vi "Send Command.vi"(8 "error in (no error)":errorcluster, 10 "command":string, 11 "GH2 in":refnum<class "GH2.lvclass">) -> (0 "error out":errorcluster, 2 "response":string, 3 "GH2 out":refnum<class "GH2.lvclass">)   [LabVIEW 2026, in "GH2.lvclass"]
uses:
  GH2.lvclass
  GH2.lvclass/GH2.ctl
  <vilib>/Utility/error.llb/Trim Whitespace One-Sided.vi
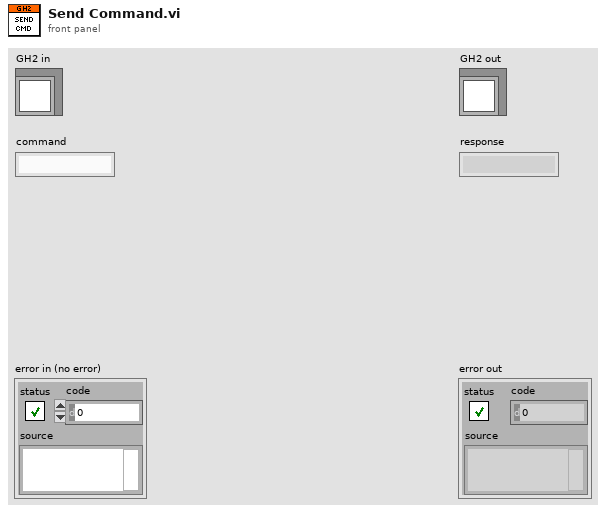
[diagram p1: front panel]
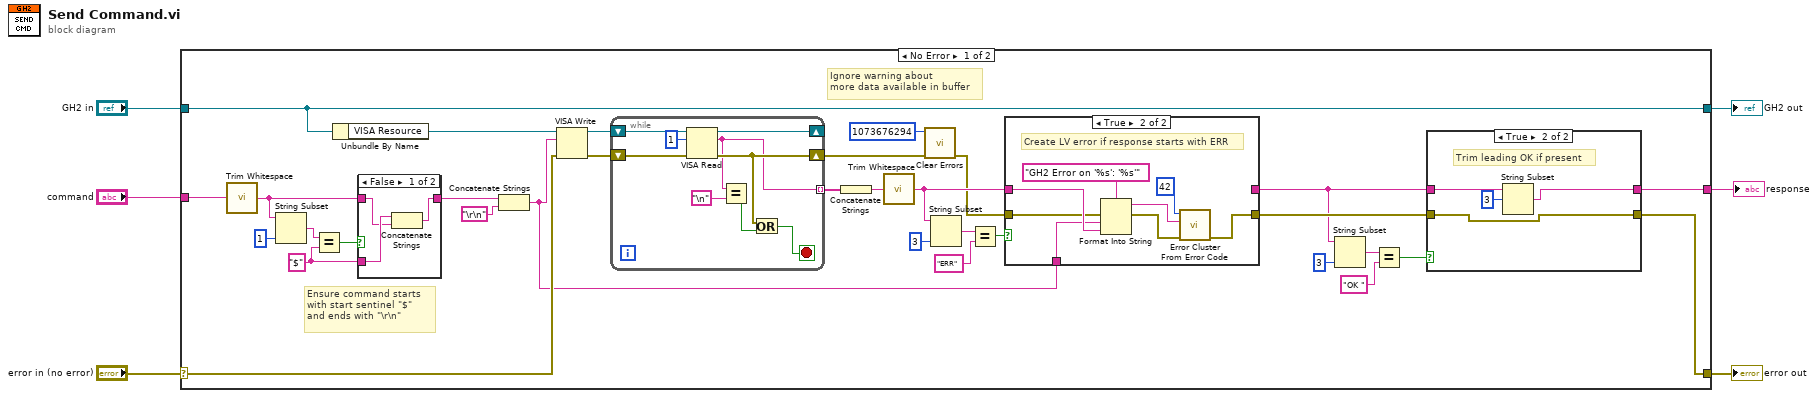
[diagram p0: block diagram]
diagram:
  n1 = case shown="No Error" "error in (no error)" {
    selector: "error in (no error)" -> [w30 w69]
    tunnel: [w7 w69] -> w5
    tunnel: [w38 w68] -> w3
    tunnel: "GH2 in" -> [w38 w68]
    tunnel: "command" -> [w37 _]
    tunnel: [w8 _] -> w1
    frame No Error {
      w32 = "$" ("y")
      # "Ignore warning about \nmore data available in buffer"
      # "Ensure command starts \nwith start sentinel \"$\" \nand ends with \"\\r\\n\""
      n2 = call <vilib>:"Trim Whitespace.vi"("string"=w37) -> ("trimmed string"=w33:string)  [unwired: 1 in]
      n3 = String Subset(string=w33, length (rest)=1 ("length (rest)")) -> (substring=w35:string)  [unwired: 1 in]
      n4 = Equal?(x=w35, y=w32) -> (x = y?=w34:bool)
      n5 = Unbundle By Name(w38) -> ("VISA Resource"=w31:refnum<visa-resource-name>)
      n6 = case shown="False" w34 {
        tunnel: w33 -> [w65 w67]
        tunnel: [w64 w67] -> w24
        tunnel: w32 -> [w66 _]
        frame False {
          n7 = Concatenate Strings(w66, w65) -> (w64:string)
        }
        frame True {
        }
      }
      n8 = Concatenate Strings(w24, "\r\n") -> (w18:string)
      n9 = VISA Write(VISA resource name=w31, write buffer=w18, error in (no error)=w30) -> (VISA resource name out=w29:refnum<visa-resource-name>, error out=w28:errorcluster)  [unwired: 1 out]
      n10 = while {
        shift-right: [w59] -> w17
        shift-left: w28 -> [w61]
        shift-right: [w60] -> _
        shift-left: w29 -> [w63]
        tunnel: [w55] -> w27 mode=indexing
        stop <- w58 stop-if-true
        n11 = VISA Read(VISA resource name=w63, byte count=u32 1, error in (no error)=w61) -> (VISA resource name out=w60:refnum<visa-resource-name>, read buffer=w55:string, error out=w59:errorcluster)  [unwired: 1 out]
        n12 = Equal?(x=w55, y="\n") -> (x = y?=w56:bool)
        n13 = Or(x=w59, y=w56) -> (x .or. y?=w58:bool)
      }
      n14 = Concatenate Strings(w27) -> (w26:string)
      n15 = call <vilib>:"Trim Whitespace.vi"("string"=w26) -> ("trimmed string"=w20:string)  [unwired: 1 in]
      n16 = call <vilib>:"Clear Errors.vi"("error in (no error)"=w17, "specific error code to clear (0: all)"=1073676294) -> ("error out"=w16:errorcluster)  [unwired: 4 in, 1 out]
      n17 = String Subset(string=w20, length (rest)=3 ("length (rest)")) -> (substring=w22:string)  [unwired: 1 in]
      n18 = Equal?(x=w22, y="ERR") -> (x = y?=w19:bool)
      n19 = case shown="True" w19 {
        tunnel: w20 -> [w46 w53]
        tunnel: [w46 _] -> w9
        tunnel: w16 -> [w45 w50]
        tunnel: [w45 w48] -> w10
        tunnel: w18 -> [_ w47]
        frame False {
        }
        frame True {
          # "Create LV error if response starts with ERR"
          n20 = Format Into String(format string="GH2 Error on '%s': '%s'", error in=w50, w47, w53) -> (resulting string=w52:string, error out=w49:errorcluster)  [unwired: 1 in]
          n21 = call <vilib>:"Error Cluster From Error Code.vi"("error in (no error)"=w49, "error message (\"\")"=w52, "error code (0)"=42) -> ("error out"=w48:errorcluster)  [unwired: 6 in]
        }
      }
      n22 = String Subset(string=w9, length (rest)=3 ("length (rest)")) -> (substring=w13:string)  [unwired: 1 in]
      n23 = Equal?(x=w13, y="OK ") -> (x = y?=w11:bool)
      n24 = case shown="True" w11 {
        tunnel: w9 -> [w39 w44]
        tunnel: w10 -> [w40 w42]
        tunnel: [w40 w42] -> w7
        tunnel: [w39 w41] -> w8
        frame False {
        }
        frame True {
          # "Trim leading OK if present"
          n25 = String Subset(string=w44, offset (0)=3) -> (substring=w41:string)  [unwired: 1 in]
        }
      }
    }
    frame Error {
    }
  }
  "error out" <- w5
  "GH2 out" <- w3
  "response" <- w1
